vi "FGV_REWORK_connection_reference.vi"(7 "options":T1, 8 "error_in":errorcluster, 11 "reference_in":refnum<k5>) -> (0 "error_out":errorcluster, 1 "killed?":bool, 2 "connection_ID_out":refnum<k5>, 3 "listener_ID_out":refnum<k5>)   [LabVIEW 2019]
uses:
  FGV_REWORK_connection_reference.ctl
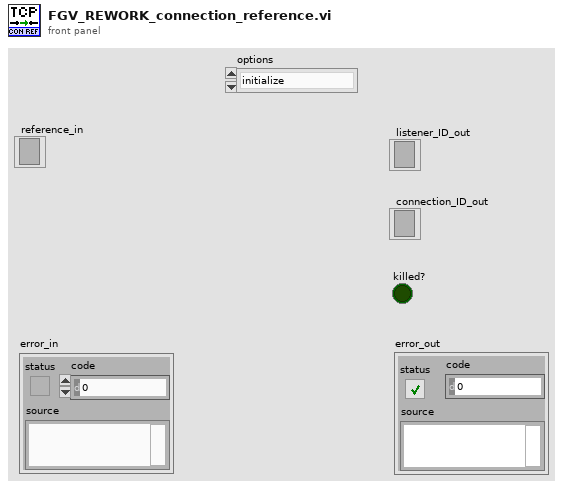
[diagram p1: front panel]
types:
  T1 = typedef "FGV_REWORK_connection_reference.ctl" = enum16{"initialize", "set_listener_ID", "set_connection_ID", "get", "KILL_ALL_CONNECTIONS", "killed?"}
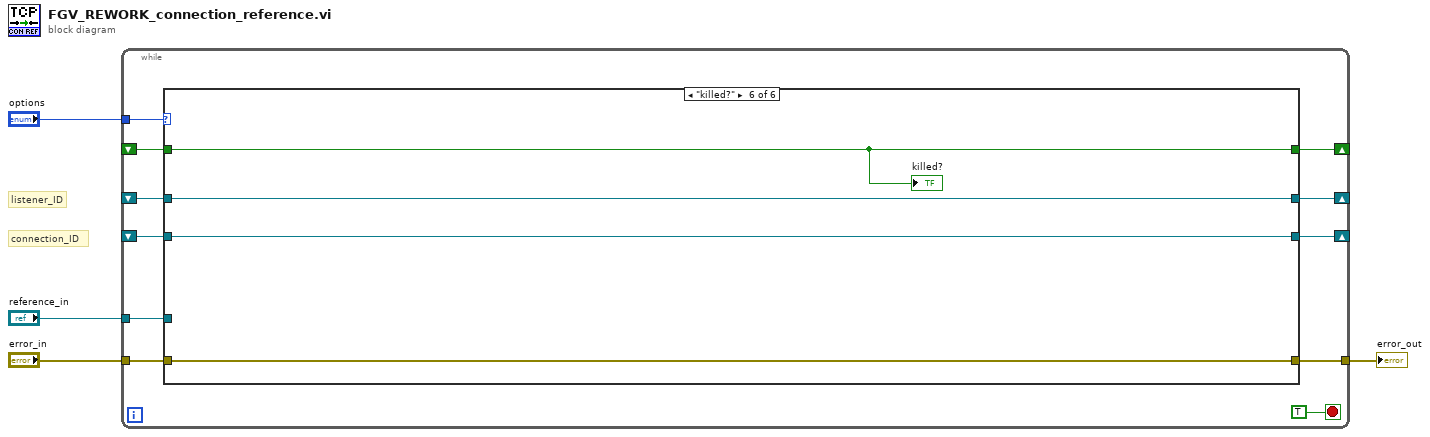
[diagram p0: block diagram]
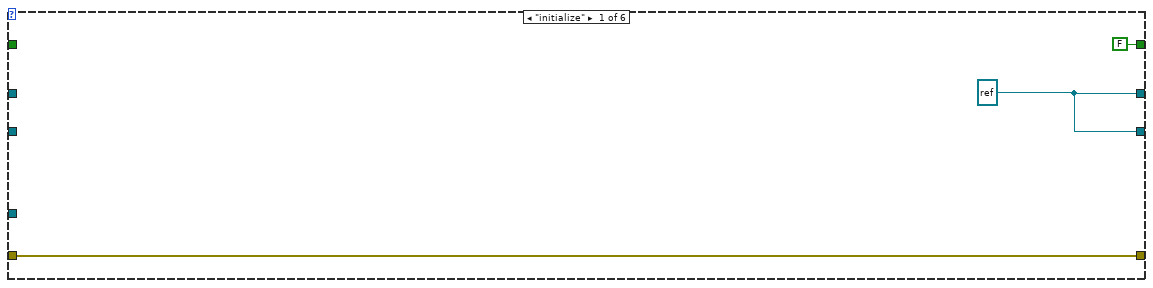
[diagram p2: hidden frame]
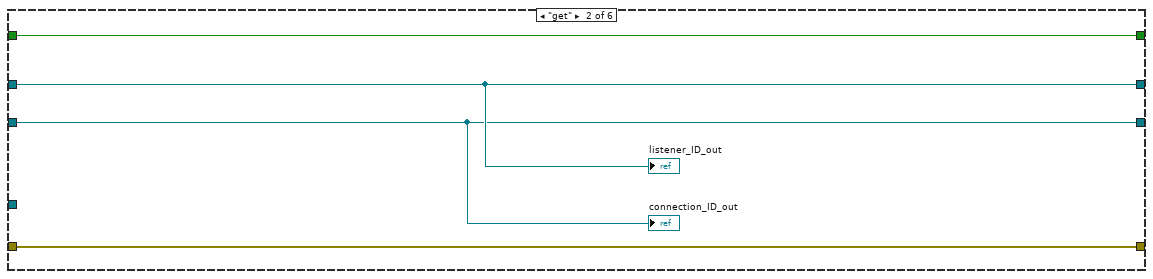
[diagram p3: hidden frame]
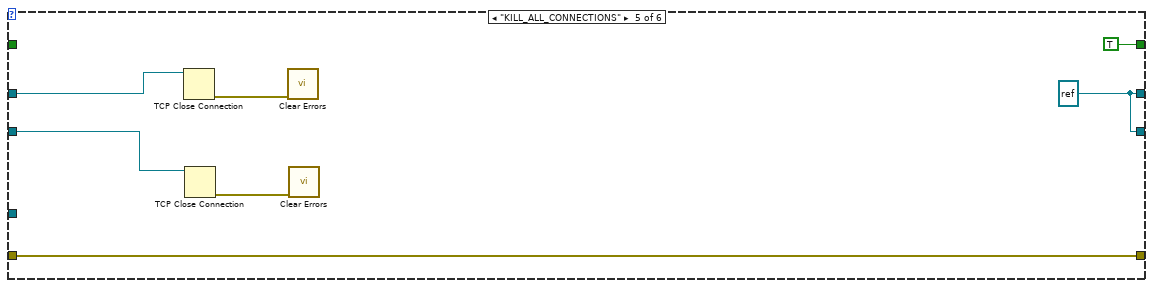
[diagram p6: hidden frame]
diagram:
  # "connection_ID"
  # "listener_ID"
  n1 = while {
    tunnel: "options" -> [w14]
    tunnel: [w13] -> w4
    tunnel: "error_in" -> [w12]
    shift-right: [w11] -> _
    shift-left: _ -> [w9]
    tunnel: "reference_in" -> [w10]
    shift-right: [w8] -> _
    shift-left: _ -> [w7]
    shift-right: [w6] -> _
    shift-left: _ -> [w5]
    stop <- TRUE stop-if-true
    n2 = case shown="\"killed?\"" w14 {
      tunnel: [w18 w22 w26 w30 w37 w39] -> w13
      tunnel: w12 -> [w18 w22 w26 w30 w37 w39]
      tunnel: [w16 w20 w23 w29 w31 w41] -> w11
      tunnel: w9 -> [_ w20 _ w29 w36 w41]
      tunnel: w10 -> [_ _ w23 w27 _ _]
      tunnel: [w16 w19 w25 w27 w31 w40] -> w8
      tunnel: w7 -> [_ w19 w25 _ w33 w40]
      tunnel: [FALSE w21 w24 w28 TRUE w38] -> w6
      tunnel: w5 -> [_ w21 w24 w28 _ w38]
      frame "initialize" {
        w16 = refnum<k5> refnum ("connection ID")
      }
      frame "get" {
        "listener_ID_out" <- w20
        "connection_ID_out" <- w19
      }
      frame "set_listener_ID" {
      }
      frame "set_connection_ID" {
      }
      frame "KILL_ALL_CONNECTIONS" {
        w31 = refnum<k5> refnum ("connection ID")
        n3 = TCP Close Connection(connection ID=w36) -> (error out=w35:errorcluster)  [unwired: 2 in, 1 out]
        n4 = TCP Close Connection(connection ID=w33) -> (error out=w34:errorcluster)  [unwired: 2 in, 1 out]
        n5 = call <vilib>:"Clear Errors.vi"("error in (no error)"=w35) -> ()  [unwired: 5 in, 2 out]
        n6 = call <vilib>:"Clear Errors.vi"("error in (no error)"=w34) -> ()  [unwired: 5 in, 2 out]
      }
      frame "killed?" {
        "killed?" <- w38
      }
    }
  }
  "error_out" <- w4
